vi "Parse Core(override).vi"(8 "error in (no error)":errorcluster, 11 "QPA TCF Parser in":refnum<class "QPA TCF Parser.lvclass">) -> (0 "error out":errorcluster, 2 "Dictionaries Out":refnum<class "String Database.lvclass">[](array[class]), 3 "QPA TCF Parser out":refnum<class "QPA TCF Parser.lvclass">)   [LabVIEW 2016, in "QPA TCF Parser.lvlib" / "QPA TCF Parser.lvclass"]
uses:
  QPA TCF Parser.lvclass
  C:/Projects/STS/Common/Sequence Automation/Plugins/File Parsing Interface.lvlibp/File Parsing Interface.lvclass
  Plugins/String Database.lvlibp/String Database.lvclass
  Plugins/File Parsing Interface.lvlibp/Accessors/File to Parse/Read File to Parse.vi
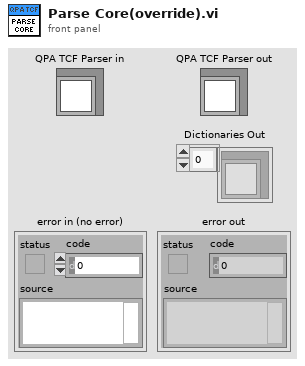
[diagram p1: front panel]
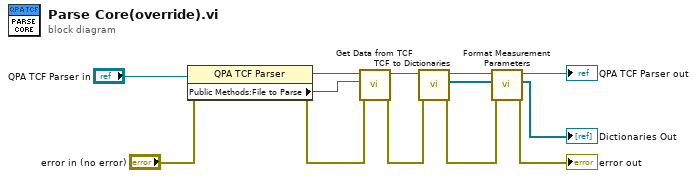
[diagram p0: block diagram]
diagram:
  n1 = property class="QPA TCF Parser"(reference="QPA TCF Parser in", error in="error in (no error)") -> (reference out=w9:refnum<class "QPA TCF Parser.lvclass">, error out=w11:errorcluster, "Public Methods:File to Parse"=w8:path)
  n2 = call "Get Data from TCF.vi"("error in (no error)"=w11, "TCF Path"=w8, "QFE3320 TCF Parser in"=w9) -> ("error out"=w12:errorcluster, "QFE3320 TCF Parser out"=w6:refnum<class "QPA TCF Parser.lvclass">)  [unwired: 7 in]
  n3 = call "TCF to Dictionaries.vi"("error in (no error)"=w12, "QPA TCF Parser in"=w6) -> ("error out"=w7:errorcluster, "Dictionaries Out"=w2:refnum<class "String Database.lvclass">[], "QPA TCF Parser out"=w4:refnum<class "QPA TCF Parser.lvclass">)  [unwired: 7 in]
  n4 = call "Format Measurement Parameters.vi"("error in (no error)"=w7, "Measurement Parameters In"=w2, "QPA TCF Parser in"=w4) -> ("error out"=→"error out":errorcluster, "Measurement Parameters Out"=→"Dictionaries Out":refnum<class "String Database.lvclass">[], "QPA TCF Parser out"=→"QPA TCF Parser out":refnum<class "QPA TCF Parser.lvclass">)  [unwired: 6 in]
